vi "MGI Shift Array (DBL[]).vi"(1 "Double[]":dbl[](array[numeric]) format="%.2f", 2 "Shift":i32) -> (0 "Shifted Double[]":dbl[](array[numeric]) format="%.2f")   [LabVIEW 2016]
doc: "Shift a double precision 1-D array by a specified amount up or down, filling with NaN.\n\nAuthored by David A. Moore\nsupport@mooregoodideas.com\nwww.mooregoodideas.com\n\nCopyright (c) 2010, Moore Good Ideas, Inc.\n\nAll rights reserved.\n\nRedistribution and use in source and binary forms, with or without modification, are permitted provided that the following conditions are met:\n\n * Redistributions of source code must retain the above copyright notice, this list of conditions and the following disclaimer.\n * Redistributions in binary form must reproduce the above copyright notice, this list of conditions and the following disclaimer in the documentation and/or other materials provided with the distribution.\n * Neither the name of Moore Good Ideas, Inc. nor the names of its contributors may be used to endorse or promote products derived from this software without specific prior written permission.\n\nTHIS SOFTWARE IS PROVIDED BY THE COPYRIGHT HOLDERS AND CONTRIBUTORS \"AS IS\" AND ANY EXPRESS OR IMPLIED WARRANTIES, INCLUDING, BUT NOT LIMITED TO, THE IMPLIED WARRANTIES OF MERCHANTABILITY AND FITNESS FOR A PARTICULAR PURPOSE ARE DISCLAIMED. IN NO EVENT SHALL THE COPYRIGHT OWNER OR CONTRIBUTORS BE LIABLE FOR ANY DIRECT, INDIRECT, INCIDENTAL, SPECIAL, EXEMPLARY, OR CONSEQUENTIAL DAMAGES (INCLUDING, BUT NOT LIMITED TO, PROCUREMENT OF SUBSTITUTE GOODS OR SERVICES; LOSS OF USE, DATA, OR PROFITS; OR BUSINESS INTERRUPTION) HOWEVER CAUSED AND ON ANY THEORY OF LIABILITY, WHETHER IN CONTRACT, STRICT LIABILITY, OR TORT (INCLUDING NEGLIGENCE OR OTHERWISE) ARISING IN ANY WAY OUT OF THE USE OF THIS SOFTWARE, EVEN IF ADVISED OF THE POSSIBILITY OF SUCH DAMAGE."
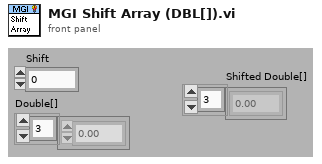
[diagram p1: front panel]
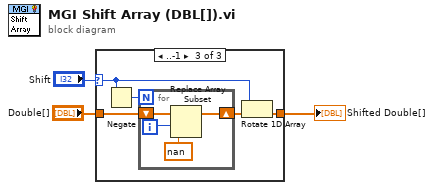
[diagram p0: block diagram]
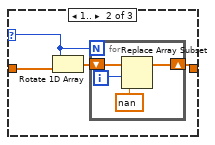
[diagram p3: hidden frame]
diagram:
  n1 = case shown="..-1" "Shift" {
    selector: "Shift" -> [_ w7 w15]
    tunnel: "Double[]" -> [w4 w8 w17]
    tunnel: [w4 w5 w14] -> w1
    frame 0 {
    }
    frame 1.. {
      n2 = Rotate 1D Array(1:w8, 2:w7) -> (0:w6:dbl[])
      n3 = for {
        N: w7 -> [_]
        shift-right: [w9] -> w5
        shift-left: w6 -> [w12]
        i -> [w11]
        n4 = Replace Array Subset(array=w12, new element=nan ("New Element/Subarray"), index=w11) -> (w9:dbl[])
      }
    }
    frame ..-1 {
      n5 = Negate(x=w15) -> (-x=w13:i32)
      n6 = for {
        N: w13 -> [_]
        shift-right: [w18] -> w16
        shift-left: w17 -> [w21]
        i -> [w20]
        n7 = Replace Array Subset(array=w21, new element=nan ("New Element/Subarray"), index=w20) -> (w18:dbl[])
      }
      n8 = Rotate 1D Array(1:w16, 2:w15) -> (0:w14:dbl[])
    }
  }
  "Shifted Double[]" <- w1
